vi "Get_Call_chain.vi"(0 "Message":string) -> (1 "Output String":string, 2 "VI to open":string)   [LabVIEW 2010]
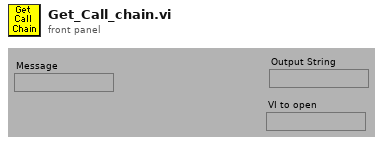
[diagram p1: front panel]
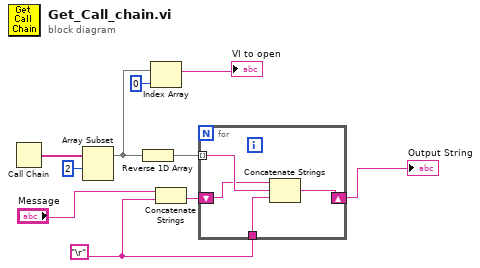
[diagram p0: block diagram]
diagram:
  w3 = "\r"
  n1 = Call Chain() -> (call chain=w8:string[])
  n2 = Array Subset(array=w8, index=2) -> (w5:string[])  [unwired: 1 in]
  n3 = Reverse 1D Array(array=w5) -> (reversed array=w7:string[])
  n4 = Index Array(array=w5, index=0) -> (element=→"VI to open":string)
  n5 = Concatenate Strings("Message", w3) -> (w10:string)
  n6 = for {
    shift-right: [w12] -> w2
    shift-left: w10 -> [w13]
    tunnel: w7 -> [w14] mode=indexing
    tunnel: w3 -> [w11]
    n7 = Concatenate Strings(w13, w14, w11) -> (w12:string)
  }
  "Output String" <- w2
